vi "Тест_буфера_дублирвание_строк.vi"() -> ()   [LabVIEW 2017]
panel:
  out "Array 2":dbl[](array[numeric])
  out "output array 3":dbl[](array[numeric])
  out "Numeric 2":dbl
  out "Numeric":dbl
  out "см. 1.5":dbl[][](array[numeric])
  in  "Кол-во копий 2":i32=5
  out "output array":dbl[](array[numeric])
  out "Исходное сообщение":dbl[](array[numeric])
  in  "Кол-во копий":i32=5
  out "Подготовленный к отправке мажоритарный код":dbl[][](array[numeric])
  out "2-х массив на выходе 3":dbl[][](array[numeric])
  in  "Размер окна":i32=4
  out "Последовательность в массиве":dbl[](array[numeric])
  in  "Кол-во элементов":i32=16
  out "Array":dbl[][](array[numeric])
  in  "Размер окна буффера":i32
  out "Количество бит":i32
  in  "Количество бит":i32=8
  out "Биты на выходе":dbl[](array[numeric])
  # "3"
  # "15"
  # "7"
  # "3"
  # "7"
  # "15"
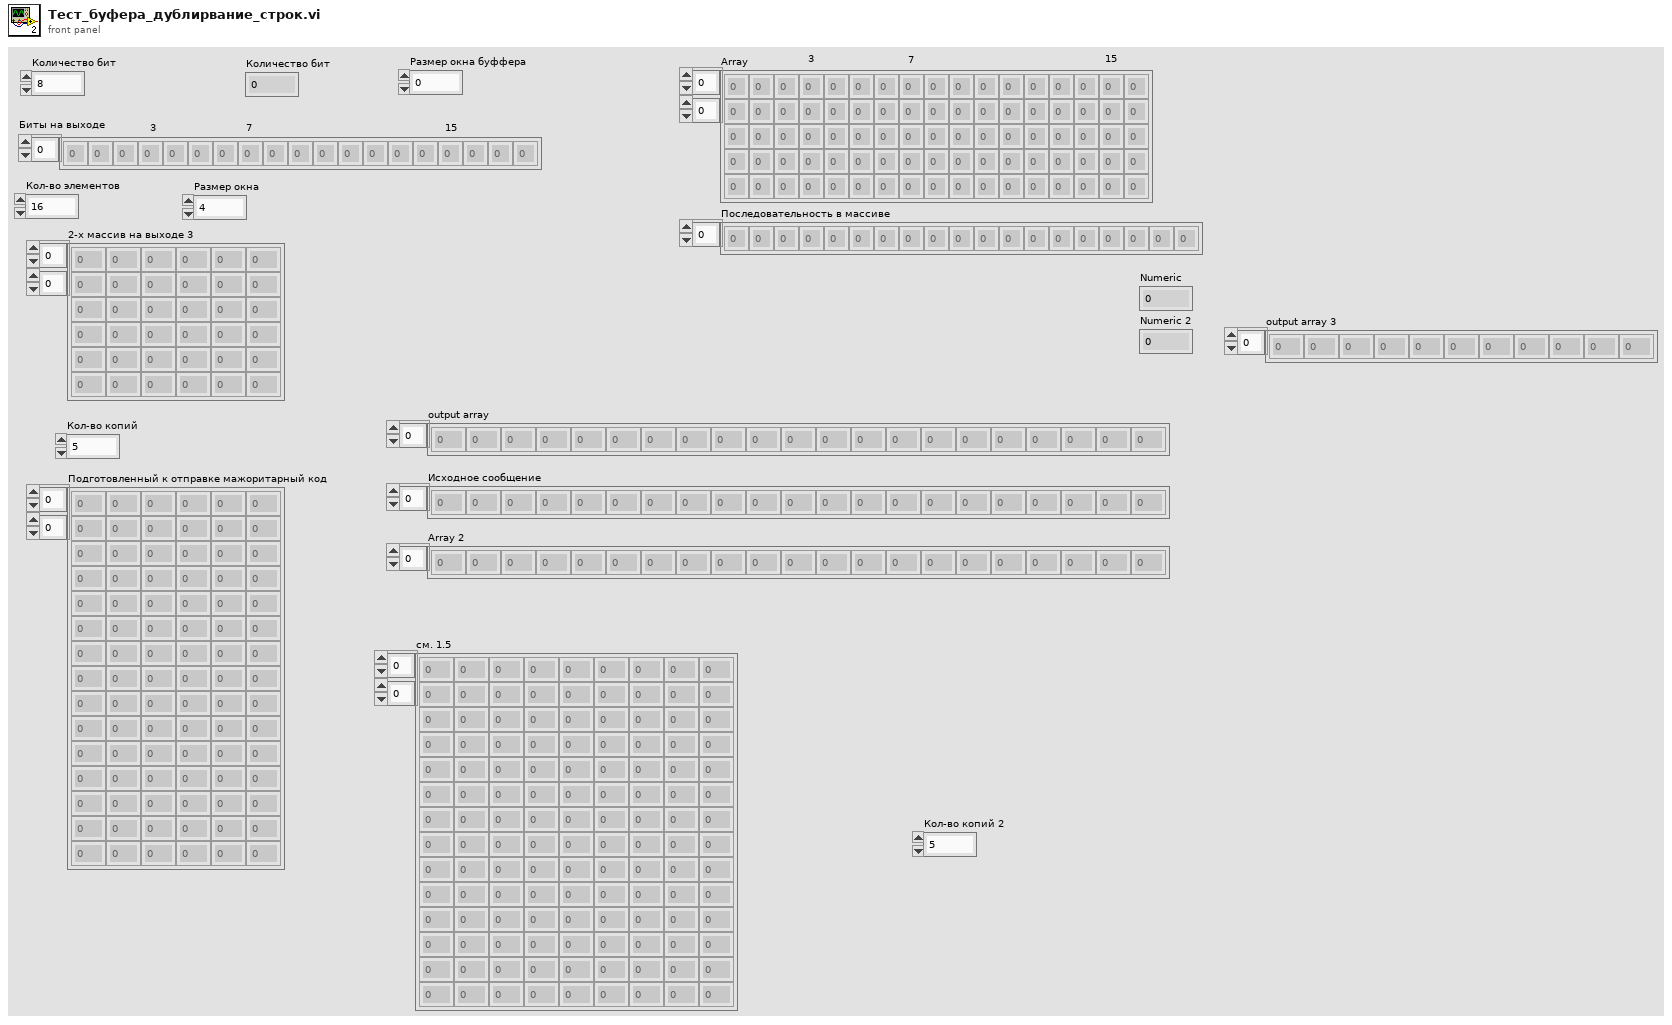
[diagram p1: front panel]
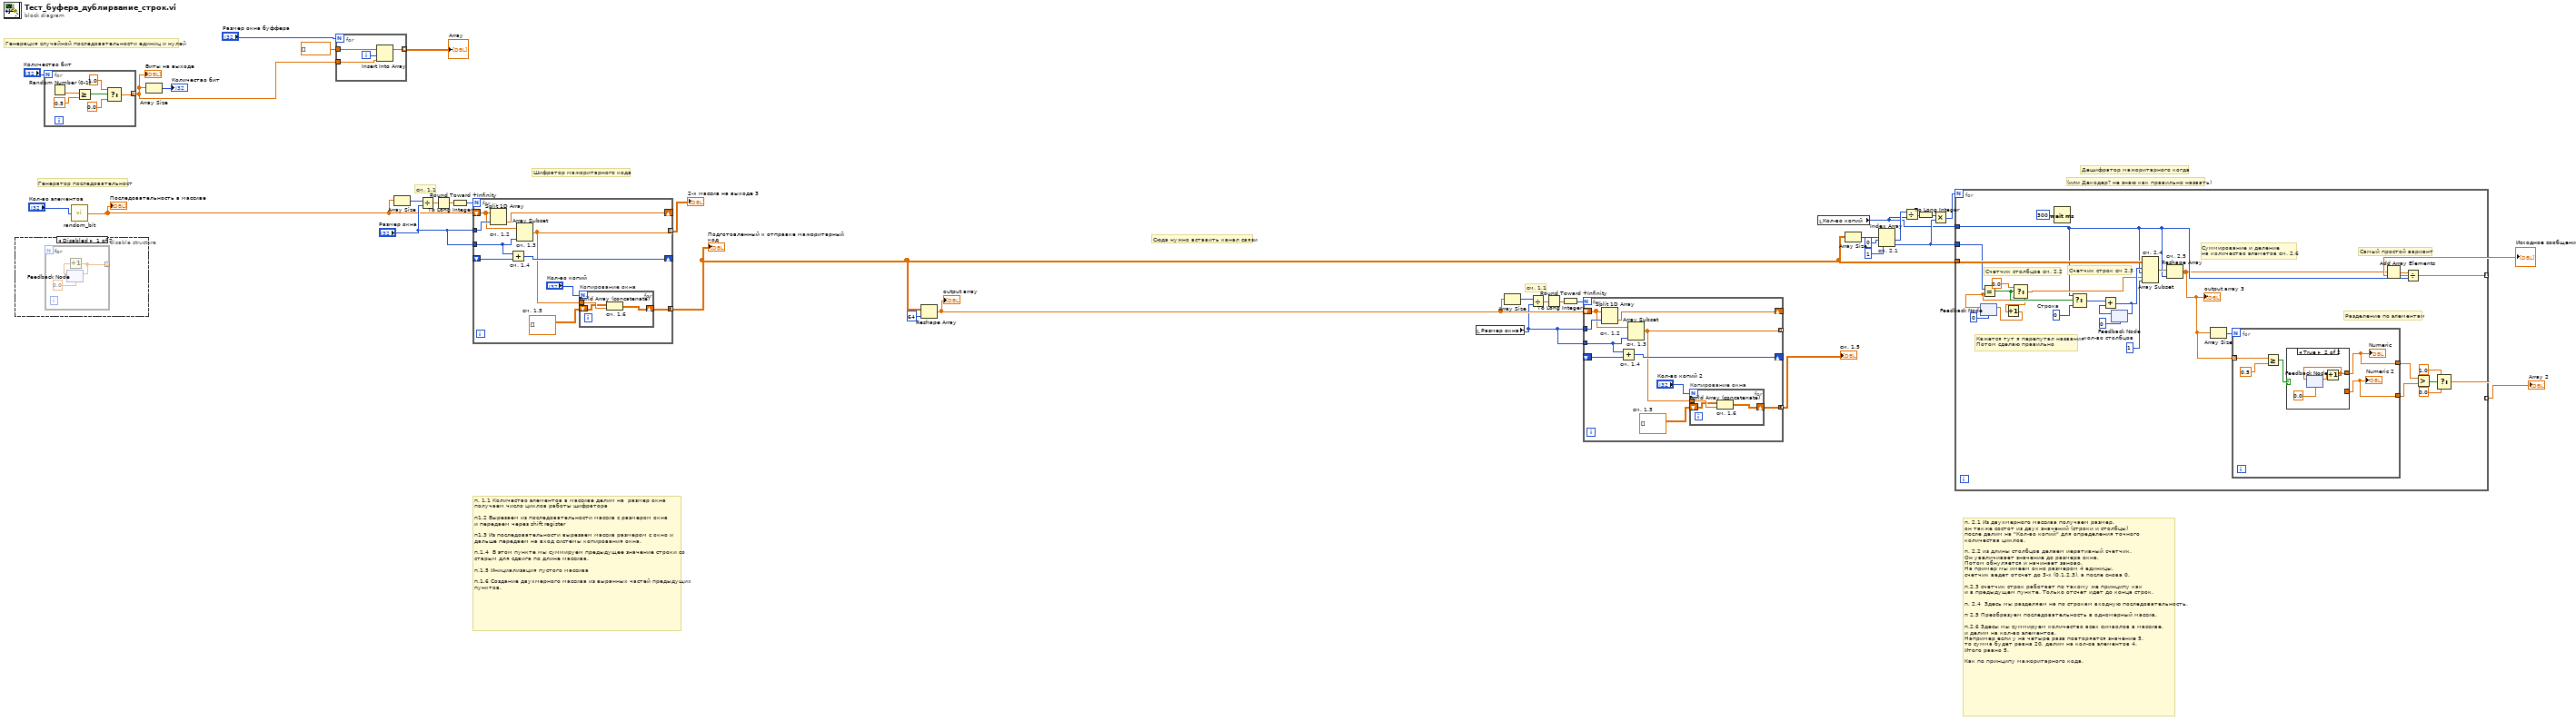
[diagram p0: block diagram]
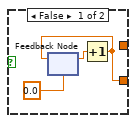
[diagram p3: hidden frame]
diagram:
  # "Сюда нужно вставить канал связи"
  # "см. 1.1"
  # "п. 2.1 Из двухмерного массива получаем размер.\nон также состот из двух значений (строки и столбцы) \nпосле делим на \"Кол-во копий\" для определения точного\nколичества циклов.\n\nп. 2.2 из длины столбцов делаем иеративный счетчик. \nОн увеличивает значение до размера окна.\nПотом обнуляется и начинает заново.\nНа пример мы имеем окно размером 4 единицы.\nсчетчик ведет отсчет до 3-х (0,1,2,3), а после снова 0.\n\nп.2.3 счетчик строк работает по такому же принципу как \nи в предыдущем пункте. Только отсчет идет до конца строк.\n\nп. 2.4  Здесь мы разделяем на по строкам входную последовательность.\n\nп 2.5 Преобразуем последовательность в одномерный массив.\n\nп.2.6 Здесы мы суммируем количество всех символов в массиве.\nи делим на кол-во элементов.\nНапример если у на четыре раза повторяется значение 5, \nто сумма будет равна 20, делим на кол-ов элементов 4. \nИтого равно 5. \n\nКак по принципу мажоритарного кода."
  # "п. 1.1 Количество элементов в массиве делим на  размер окна\nполучаем число циклов работы шифратора\n\nп1.2 Вырезаем из последовательности массив с размером окна \nи передаем через shift register\n\nп1.3 Из последовательности вырезаем массив размером с окно и \nдальше передаем на вход системы копирования окна.\n \nп.1.4  В этом пункте мы суммируем предыдущее значение строки со\nстарым для сдвига по длине массива.\n\nп.1.5 Инициализация пустого массива\n\nп.1.6 Создание двухмерного массива из выранных частей предыдущих\nпунктов."
  # "см. 1.1"
  # "(или Декодер? не знаю как правильно назвать)"
  # "Дешифратор мажоритарного когда"
  # "Шифратор мажоритарного кода"
  # "Генератор последовательност"
  # "Генерация случайной последовательности единиц и нулей"
  n1 = disable-structure shown="Disabled" {
    frame Disabled {
      n2 = for {
        tunnel: [w35] -> _ mode=indexing
        n3 = feedback #1(0.0) -> (w37:dbl)
        n4 = Increment(x=w37) -> (x+1=w35:dbl)
        n5 = feedback-in #1(w35) -> ()
      }
    }
    frame Enabled {
    }
  }
  n6 = for {
    N: "Количество бит" -> [_]
    tunnel: [w38] -> w29 mode=indexing
    n7 = Random Number (0-1)() -> (number: 0 to 1=w43:dbl)
    n8 = Greater Or Equal?(x=w43, y=0.5) -> (x >= y?=w41:bool)
    n9 = Select(t=1.0, s=w41, f=0.0) -> (s? t:f=w38:dbl)
  }
  "Биты на выходе" <- w29
  n10 = call "random_bit.vi"("Количество бит"="Кол-во элементов") -> ("Биты на выходе 1"=w2:dbl[])
  "Последовательность в массиве" <- w2
  n11 = Array Size(array=w29) -> (size(s)=→"Количество бит":i32)
  n12 = for {
    N: "Размер окна буффера" -> [_]
    tunnel: w29 -> [w45]
    tunnel: dbl[] [] -> [w46]
    tunnel: [w47] -> w32 mode=indexing
    i -> [w44]
    n13 = Insert Into Array(array=w46, index=w44, new element=w45) -> (w47:dbl[])
  }
  "Array" <- w32
  n14 = Array Size(array=w2) -> (size(s)=w28:i32)
  n15 = Divide(x=w28, y="Размер окна") -> (x/y=w27:dbl)
  n16 = Round Toward +Infinity(x=w27) -> (ceil(x): smallest int >= x=w26:dbl)
  n17 = To Long Integer(number=w26) -> (32bit integer=w23:i32)
  n18 = for {
    N: w23 -> [_]
    shift-right: [w57] -> _
    shift-left: w2 -> [w55]
    tunnel: "Размер окна" -> [w56]
    shift-right: [w53] -> _
    shift-left: _ -> [w52]
    tunnel: "Размер окна" -> [w54]
    tunnel: [w50] -> w24 mode=indexing
    tunnel: [w49] -> w12 mode=concatenating
    w48 = dbl[][] []  # см. 1.5
    n19 = Split 1D Array "см. 1.2"(array=w55, index=w56) -> (second subarray=w57:dbl[])  [unwired: 1 out]
    n20 = Add "см. 1.4"(x=w54, y=w52) -> (x+y=w53:i32)
    n21 = Array Subset "см. 1.3"(array=w55, length=w54) -> (w50:dbl[])  [unwired: 1 in]
    n22 = for "Копирование окна" {
      N: "Кол-во копий" -> [_]
      tunnel: w50 -> [w59]
      shift-right: [w60] -> w49
      shift-left: w48 -> [w58]
      n23 = Build Array (concatenate) "см. 1.6"(w58, w59) -> (w60:dbl[][])
    }
  }
  "2-х массив на выходе 3" <- w24
  "Подготовленный к отправке мажоритарный код" <- w12
  n24 = Reshape Array(w12, 64 ("dimension size")) -> (w6:dbl[])
  "output array" <- w6
  n25 = local read "Размер окна"() -> (w5:i32)
  n26 = Array Size(array=w6) -> (size(s)=w7:i32)
  n27 = Divide(x=w7, y=w5) -> (x/y=w8:dbl)
  n28 = Round Toward +Infinity(x=w8) -> (ceil(x): smallest int >= x=w9:dbl)
  n29 = To Long Integer(number=w9) -> (32bit integer=w10:i32)
  n30 = for {
    N: w10 -> [_]
    shift-right: [w70] -> _
    shift-left: w6 -> [w68]
    tunnel: w5 -> [w69]
    shift-right: [w66] -> _
    shift-left: _ -> [w65]
    tunnel: w5 -> [w67]
    tunnel: [w63] -> _ mode=indexing
    tunnel: [w62] -> w4 mode=concatenating
    w61 = dbl[][] []  # см. 1.5
    n31 = Split 1D Array "см. 1.2"(array=w68, index=w69) -> (second subarray=w70:dbl[])  [unwired: 1 out]
    n32 = Add "см. 1.4"(x=w67, y=w65) -> (x+y=w66:i32)
    n33 = Array Subset "см. 1.3"(array=w68, length=w67) -> (w63:dbl[])  [unwired: 1 in]
    n34 = for "Копирование окна" {
      N: "Кол-во копий 2" -> [_]
      tunnel: w63 -> [w72]
      shift-right: [w73] -> w62
      shift-left: w61 -> [w71]
      n35 = Build Array (concatenate) "см. 1.6"(w71, w72) -> (w73:dbl[][])
    }
  }
  "см. 1.5" <- w4
  n36 = local read "Кол-во копий"() -> (w14:i32)
  n37 = Array Size(array=w12) -> (size(s)=w22:i32[])
  n38 = Index Array "см. 2.1"(array=w22, index #1=0 ("index"), index #2=1 ("index")) -> (element #1=w19:i32, element #2=w18:i32)
  n39 = Divide(x=w19, y=w14) -> (x/y=w17:dbl)
  n40 = To Long Integer(number=w17) -> (32bit integer=w16:i32)
  n41 = Multiply(x=w16, y=w18) -> (x*y=w15:i32)
  n42 = for {
    N: w15 -> [_]
    tunnel: w12 -> [w99]
    tunnel: w18 -> [w91]
    tunnel: w14 -> [w83]
    tunnel: [w82] -> w13 mode=indexing
    tunnel: [w74] -> w1 mode=indexing
    w98 = 1  # кол-во столбцов
    w89 = 0  # Строка
    # "Разделение по элементам"
    # "Самый простой вариант"
    # "Суммирование и деление \nна количество элеметов см. 2.6"
    # "Кажется тут я перепутал названия  \nПотом сделаю правильно"
    # "Счетчик строк см 2.3"
    # "Счетчик столбцов см. 2.2"
    n43 = feedback #2(0) -> (w87:dbl)
    n44 = Equal?(x=w91, y=w87) -> (x = y?=w93:bool)
    n45 = Select(t=0.0, s=w93, f=w87) -> (s? t:f=w86:dbl)
    n46 = Increment(x=w86) -> (x+1=w85:dbl)
    n47 = feedback-in #2(w85) -> ()
    n48 = Wait (ms)(milliseconds to wait=u32 300) -> ()  [unwired: 1 out]
    n49 = Select(t=w83, s=w93, f=w89) -> (s? t:f=w90:i32)
    n50 = feedback #3(0) -> (w92:i32)
    n51 = Add(x=w90, y=w92) -> (x+y=w88:i32)
    n52 = feedback-in #3(w88) -> ()
    n53 = Array Subset "см. 2.4"(array=w99, index (row)=w88, length (row)=w83, index (col)=w86, length (col)=w98) -> (w100:dbl[][])
    n54 = Reshape Array "см. 2.5"(w100, w83) -> (w80:dbl[])
    "output array 3" <- w80
    n55 = Array Size(array=w80) -> (size(s)=w81:i32)
    n56 = for {
      N: w81 -> [_]
      tunnel: w80 -> [w103] mode=indexing
      tunnel: [w102] -> w79
      tunnel: [w101] -> w78
      n57 = Greater Or Equal?(x=w103, y=0.5) -> (x >= y?=w104:bool)
      n58 = case shown="True" w104 {
        tunnel: [_ w109] -> w102
        tunnel: [w106 _] -> w101
        frame False {
          n59 = feedback #4(0.0) -> (w107:dbl)
          n60 = Increment(x=w107) -> (x+1=w106:dbl)
          n61 = feedback-in #4(w106) -> ()
        }
        frame True {
          n62 = feedback #5(0.0) -> (w110:dbl)
          n63 = Increment(x=w110) -> (x+1=w109:dbl)
          n64 = feedback-in #5(w109) -> ()
        }
      }
      "Numeric" <- w102
      "Numeric 2" <- w101
    }
    n65 = Add Array Elements(numeric array=w80) -> (sum=w84:dbl)
    n66 = Divide(x=w84, y=w83) -> (x/y=w82:dbl)
    n67 = Greater?(x=w79, y=w78) -> (0:w77:bool)
    n68 = Select(t=1.0, s=w77, f=0.0) -> (s? t:f=w74:dbl)
  }
  "Исходное сообщение" <- w13
  "Array 2" <- w1
